vi "ISP Transformation.vi"(0 "Scene Object In":refnum<vi>, 1 "Theta B":dbl(slide) scale=-180.0..180.0, 2 "Psi B":dbl(slide) scale=-180.0..180.0, 3 "Phi B":dbl(slide) scale=-180.0..180.0, 5 "Base":refnum<vi>, 7 "Gimbal":refnum<vi>, 9 "Telescope":refnum<vi>, 11 "error in (no error)":errorcluster, 12 "Theta Initial":dbl, 13 "Psi Initial":dbl, 14 "Theta":dbl(slide) step=1.0 scale=-110.0..110.0, 15 "Psi":dbl(slide) step=1.0 scale=-110.0..110.0) -> (4 "Scene Object Out":refnum<vi>, 6 "error out":errorcluster)   [LabVIEW 2015]
uses:
  <vilib>/picture/3D Picture Control/NI_3D Picture Control.lvlib
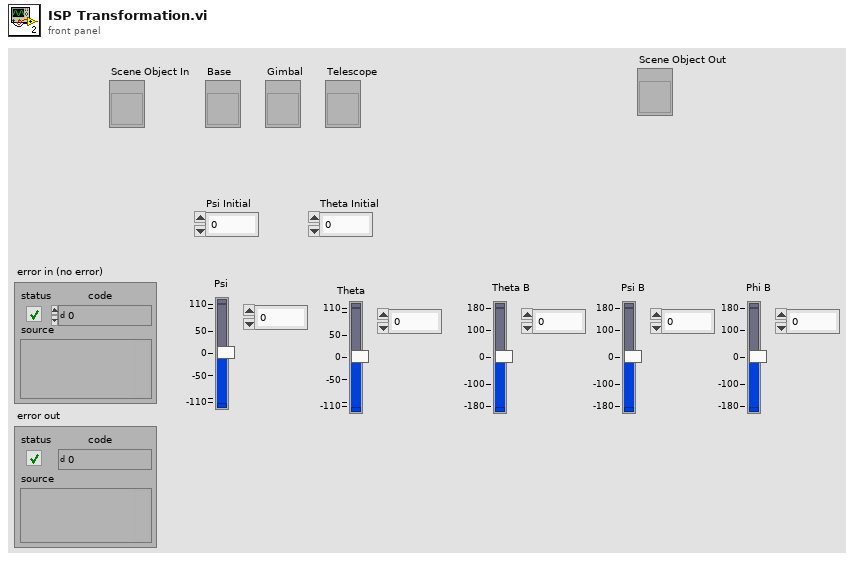
[diagram p1: front panel]
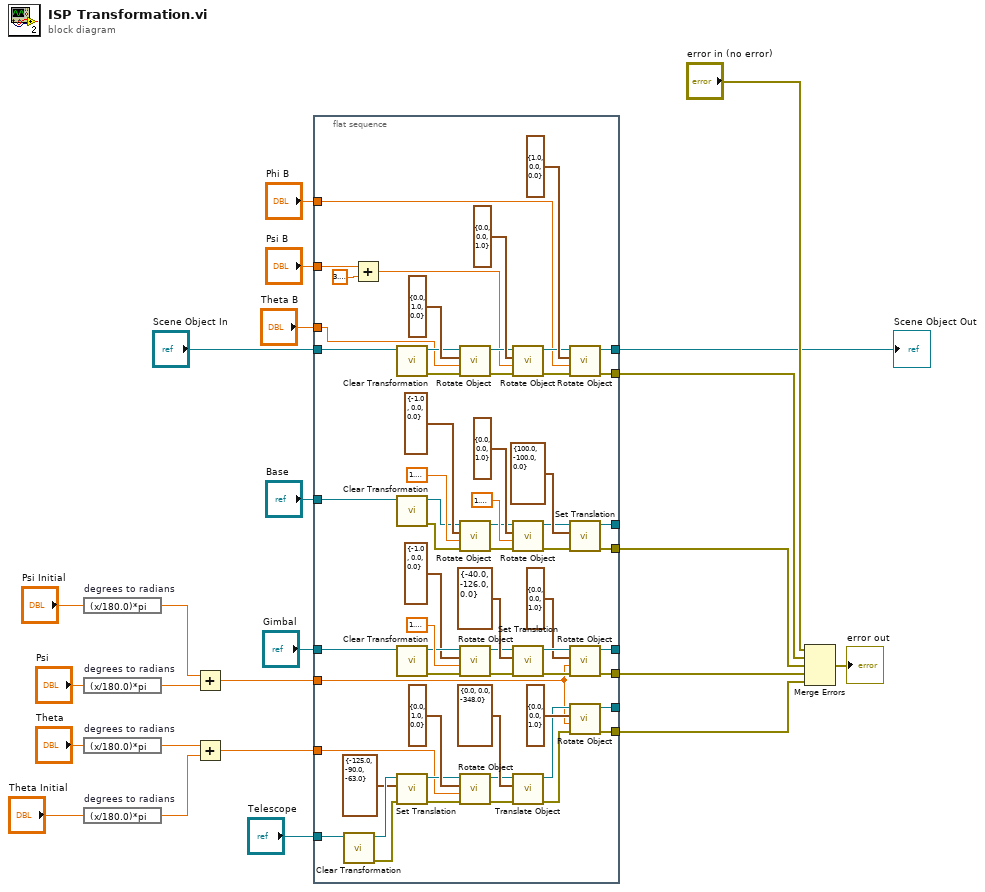
[diagram p0: block diagram]
diagram:
  n1 = expression code="(x/180.0)*pi" "degrees to radians"("Psi Initial") -> (w8:dbl)
  n2 = expression code="(x/180.0)*pi" "degrees to radians"("Psi") -> (w9:dbl)
  n3 = expression code="(x/180.0)*pi" "degrees to radians"("Theta") -> (w7:dbl)
  n4 = expression code="(x/180.0)*pi" "degrees to radians"("Theta Initial") -> (w4:dbl)
  n5 = Add(x=w8, y=w9) -> (x+y=w2:dbl)
  n6 = Add(x=w7, y=w4) -> (x+y=w3:dbl)
  n7 = flat-sequence {
    tunnel: "Telescope" -> [w84]
    tunnel: "Gimbal" -> [w83]
    tunnel: "Base" -> [w76]
    tunnel: w3 -> [w43]
    tunnel: w2 -> [w25]
    tunnel: "Scene Object In" -> [w42]
    tunnel: "Theta B" -> [w38]
    tunnel: "Psi B" -> [w26]
    tunnel: "Phi B" -> [w31]
    tunnel: [w80] -> _
    tunnel: [w79] -> w22
    tunnel: [w70] -> _
    tunnel: [w69] -> w23
    tunnel: [w51] -> _
    tunnel: [w50] -> w21
    tunnel: [w30] -> w1
    tunnel: [w29] -> w12
    frame #0 {
      n8 = call <vilib>:"Clear Transformation.vi"("Object Refnum In"=w84) -> ("error out"=w58:errorcluster, "Object Refnum Out"=w59:refnum<vi>)  [unwired: 1 in, 8 out]
      n9 = Add(x=w26, y=3.141592653589793) -> (x+y=w27:dbl)
      n10 = call <vilib>:"Clear Transformation.vi"("Object Refnum In"=w42) -> ("error out"=w39:errorcluster, "Object Refnum Out"=w40:refnum<vi>)  [unwired: 1 in, 8 out]
      n11 = call <vilib>:"Clear Transformation.vi"("Object Refnum In"=w76) -> ("error out"=w72:errorcluster, "Object Refnum Out"=w73:refnum<vi>)  [unwired: 1 in, 8 out]
      n12 = call <vilib>:"Clear Transformation.vi"("Object Refnum In"=w83) -> ("error out"=w66:errorcluster, "Object Refnum Out"=w67:refnum<vi>)  [unwired: 1 in, 8 out]
      n13 = call <vilib>:"Set Translation.vi"("error in (no error)"=w58, "Translation"=cluster{"X":sgl, "Y":sgl, "Z":sgl} {"X"=-125.0, "Y"=-90.0, "Z"=-63.0} ("Translation T1"), "Scene Object"=w59) -> ("error out"=w56:errorcluster, "Translated Object"=w57:refnum<vi>)  [unwired: 7 in]
      n14 = call <vilib>:"Rotate Object.vi"("error in (no error)"=w39, "Angle"=w38, "Axis"=cluster{"X":sgl, "Y":sgl, "Z":sgl} {"X"=0.0, "Y"=1.0, "Z"=0.0}, "Scene.Object In"=w40) -> ("error out"=w35:errorcluster, "Scene.Object Out"=w36:refnum<vi>)  [unwired: 6 in]
      n15 = call <vilib>:"Rotate Object.vi"("error in (no error)"=w72, "Angle"=1.5707963267948966, "Axis"=cluster{"X":sgl, "Y":sgl, "Z":sgl} {"X"=-1.0, "Y"=0.0, "Z"=0.0}, "Scene.Object In"=w73) -> ("error out"=w46:errorcluster, "Scene.Object Out"=w47:refnum<vi>)  [unwired: 6 in]
      n16 = call <vilib>:"Rotate Object.vi"("error in (no error)"=w66, "Angle"=1.5707963267948966, "Axis"=cluster{"X":sgl, "Y":sgl, "Z":sgl} {"X"=-1.0, "Y"=0.0, "Z"=0.0}, "Scene.Object In"=w67) -> ("error out"=w64:errorcluster, "Scene.Object Out"=w65:refnum<vi>)  [unwired: 6 in]
      n17 = call <vilib>:"Rotate Object.vi"("error in (no error)"=w56, "Angle"=w43, "Axis"=cluster{"X":sgl, "Y":sgl, "Z":sgl} {"X"=0.0, "Y"=1.0, "Z"=0.0}, "Scene.Object In"=w57) -> ("error out"=w60:errorcluster, "Scene.Object Out"=w61:refnum<vi>)  [unwired: 6 in]
      n18 = call <vilib>:"Rotate Object.vi"("error in (no error)"=w35, "Angle"=w27, "Axis"=cluster{"X":sgl, "Y":sgl, "Z":sgl} {"X"=0.0, "Y"=0.0, "Z"=1.0}, "Scene.Object In"=w36) -> ("error out"=w33:errorcluster, "Scene.Object Out"=w32:refnum<vi>)  [unwired: 6 in]
      n19 = call <vilib>:"Rotate Object.vi"("error in (no error)"=w46, "Angle"=1.5707963267948966, "Axis"=cluster{"X":sgl, "Y":sgl, "Z":sgl} {"X"=0.0, "Y"=0.0, "Z"=1.0}, "Scene.Object In"=w47) -> ("error out"=w44:errorcluster, "Scene.Object Out"=w45:refnum<vi>)  [unwired: 6 in]
      n20 = call <vilib>:"Set Translation.vi"("error in (no error)"=w64, "Translation"=cluster{"X":sgl, "Y":sgl, "Z":sgl} {"X"=-40.0, "Y"=-126.0, "Z"=0.0} ("Translation G"), "Scene Object"=w65) -> ("error out"=w81:errorcluster, "Translated Object"=w82:refnum<vi>)  [unwired: 7 in]
      n21 = call <vilib>:"Translate Object.vi"("error in (no error)"=w60, "Translation"=cluster{"X":sgl, "Y":sgl, "Z":sgl} {"X"=0.0, "Y"=0.0, "Z"=-348.0} ("Translation T2"), "Scene.Object In"=w61) -> ("error out"=w52:errorcluster, "Scene.Object Out"=w53:refnum<vi>)  [unwired: 7 in]
      n22 = call <vilib>:"Rotate Object.vi"("error in (no error)"=w33, "Angle"=w31, "Axis"=cluster{"X":sgl, "Y":sgl, "Z":sgl} {"X"=1.0, "Y"=0.0, "Z"=0.0}, "Scene.Object In"=w32) -> ("error out"=w29:errorcluster, "Scene.Object Out"=w30:refnum<vi>)  [unwired: 6 in]
      n23 = call <vilib>:"Set Translation.vi"("error in (no error)"=w44, "Translation"=cluster{"X":sgl, "Y":sgl, "Z":sgl} {"X"=100.0, "Y"=-100.0, "Z"=0.0}, "Scene Object"=w45) -> ("error out"=w69:errorcluster, "Translated Object"=w70:refnum<vi>)  [unwired: 7 in]
      n24 = call <vilib>:"Rotate Object.vi"("error in (no error)"=w81, "Angle"=w25, "Axis"=cluster{"X":sgl, "Y":sgl, "Z":sgl} {"X"=0.0, "Y"=0.0, "Z"=1.0}, "Scene.Object In"=w82) -> ("error out"=w79:errorcluster, "Scene.Object Out"=w80:refnum<vi>)  [unwired: 6 in]
      n25 = call <vilib>:"Rotate Object.vi"("error in (no error)"=w52, "Angle"=w25, "Axis"=cluster{"X":sgl, "Y":sgl, "Z":sgl} {"X"=0.0, "Y"=0.0, "Z"=1.0}, "Scene.Object In"=w53) -> ("error out"=w50:errorcluster, "Scene.Object Out"=w51:refnum<vi>)  [unwired: 6 in]
    }
  }
  n26 = Merge Errors("error in (no error)", w12, w23, w22, w21) -> (→"error out":errorcluster)
  "Scene Object Out" <- w1
